vi "equationCalculator.vi"(4 "Time Period":i8, 5 "Max profiles":T1, 6 "startOfTimePeriod":dbl, 7 "derivitave":i8, 8 "aInital (only needed for T0)":dbl, 9 "vInital":dbl, 10 "xInital":dbl, 11 "currentTime":dbl) -> (3 "output variable":dbl)   [LabVIEW 2014]
uses:
  Max profiles.ctl
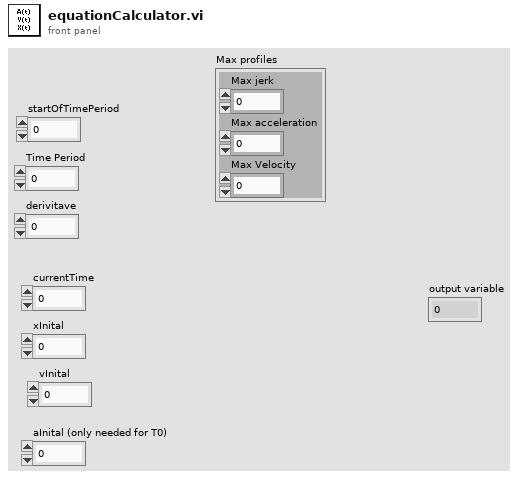
[diagram p1: front panel]
types:
  T1 = typedef "Max profiles.ctl" = cluster{"Max jerk":dbl, "Max acceleration":dbl, "Max Velocity":dbl}
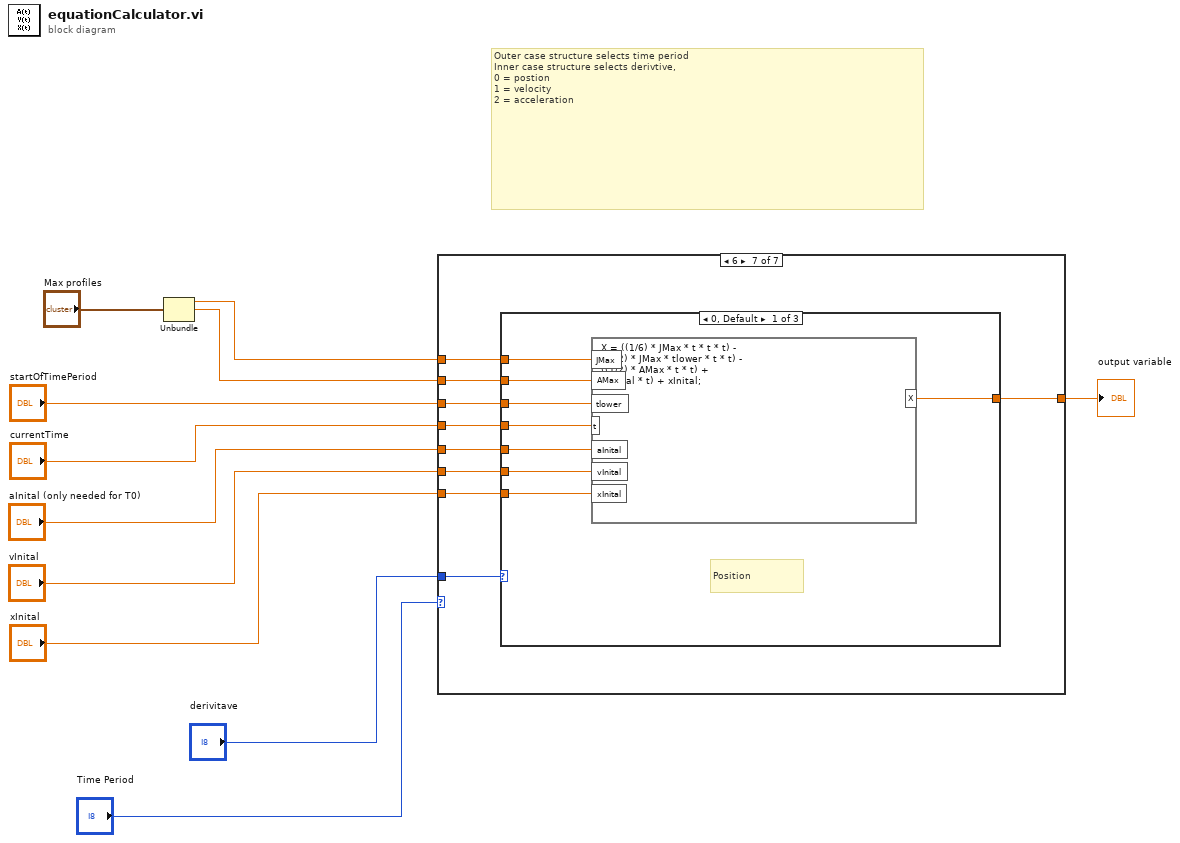
[diagram p0: block diagram]
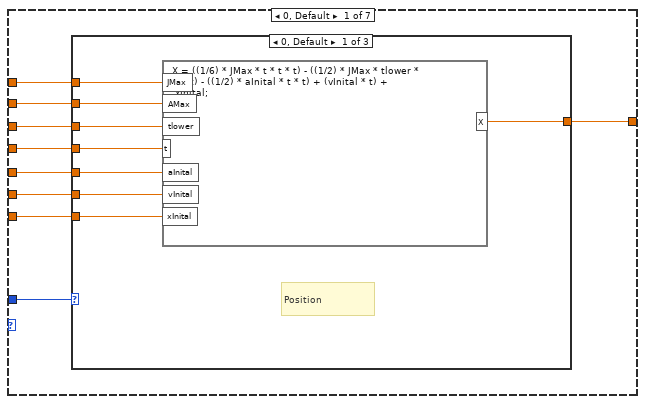
[diagram p2: hidden frame]
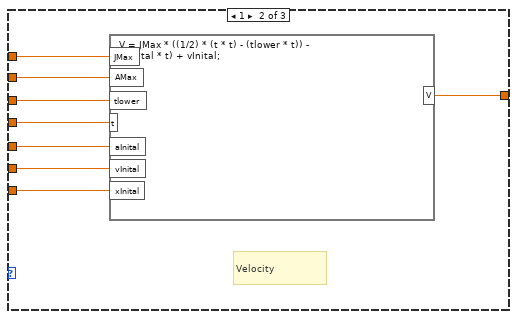
[diagram p3: hidden frame]
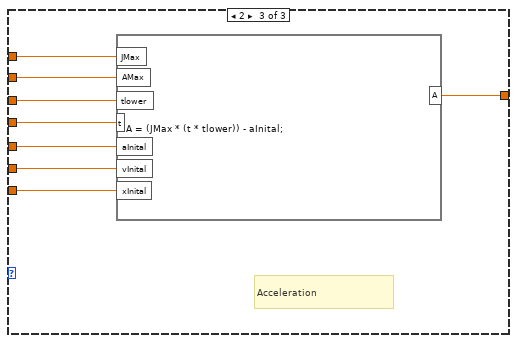
[diagram p4: hidden frame]
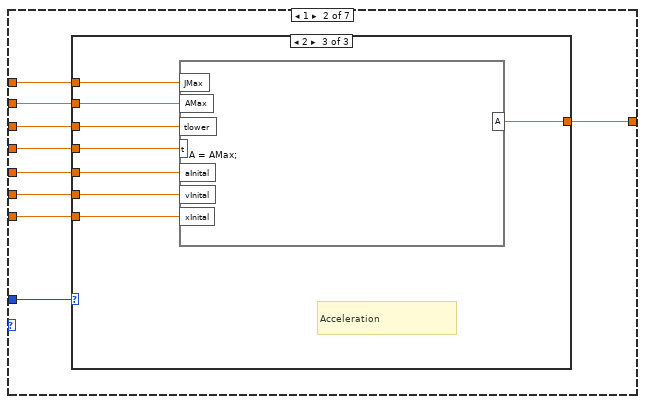
[diagram p5: hidden frame]
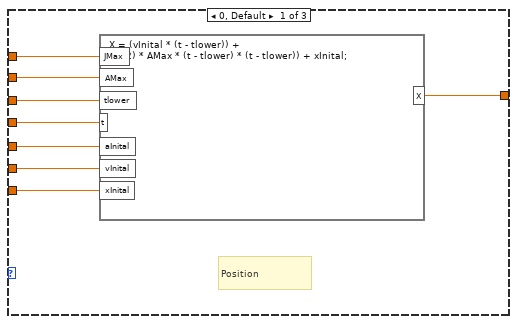
[diagram p6: hidden frame]
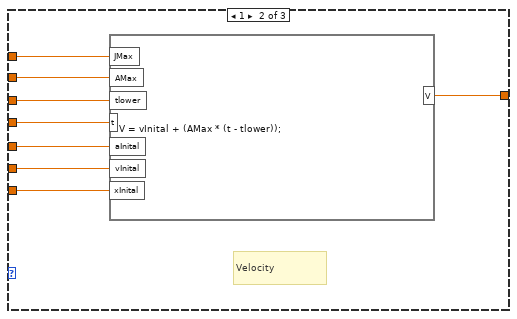
[diagram p7: hidden frame]
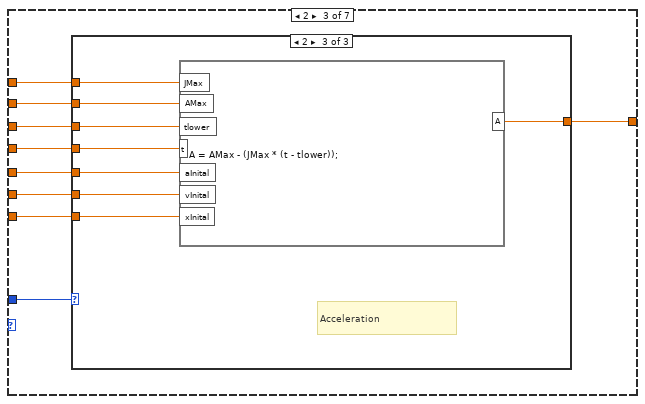
[diagram p8: hidden frame]
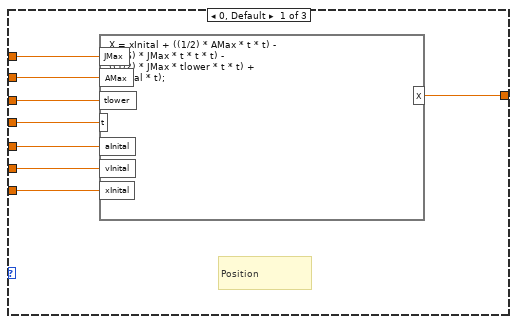
[diagram p9: hidden frame]
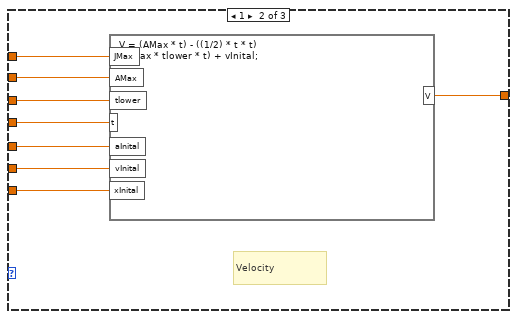
[diagram p10: hidden frame]
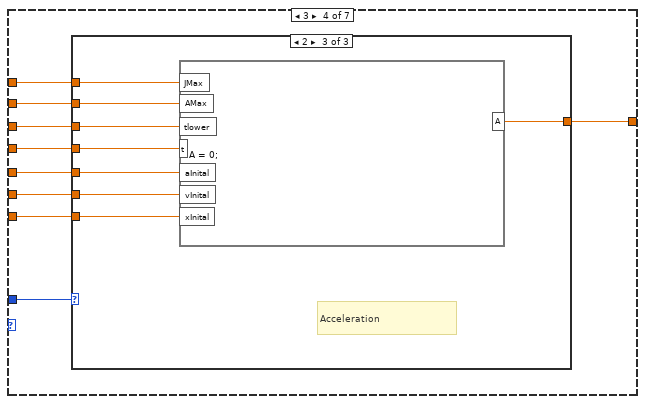
[diagram p11: hidden frame]
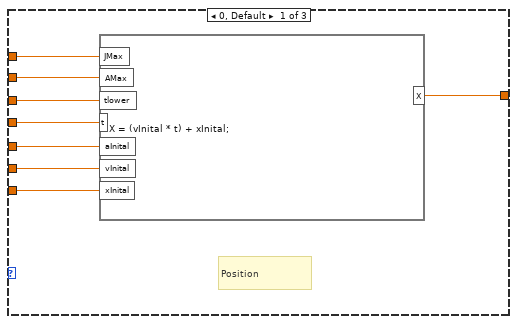
[diagram p12: hidden frame]
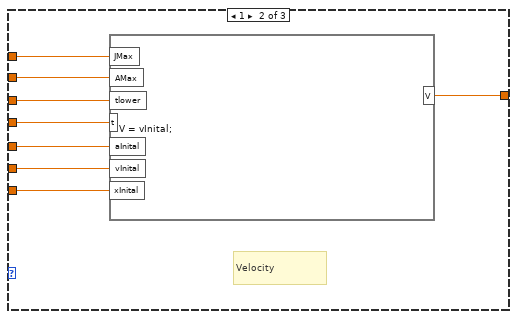
[diagram p13: hidden frame]
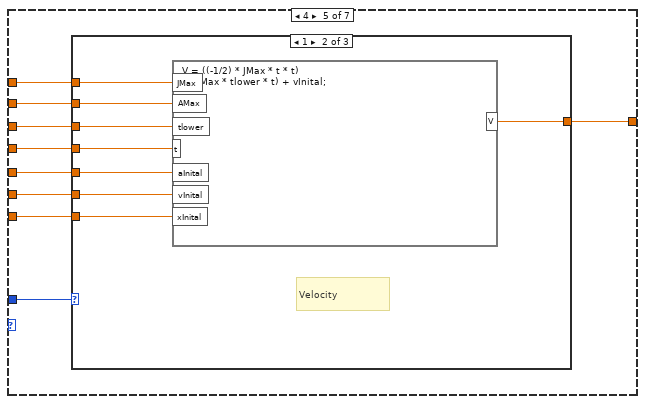
[diagram p14: hidden frame]
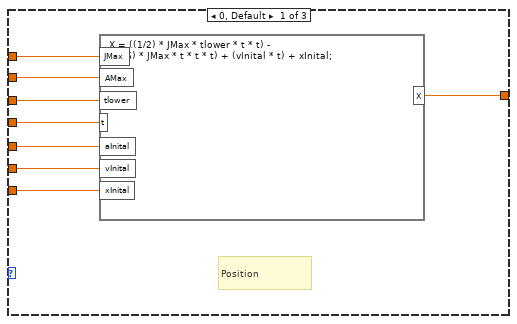
[diagram p15: hidden frame]
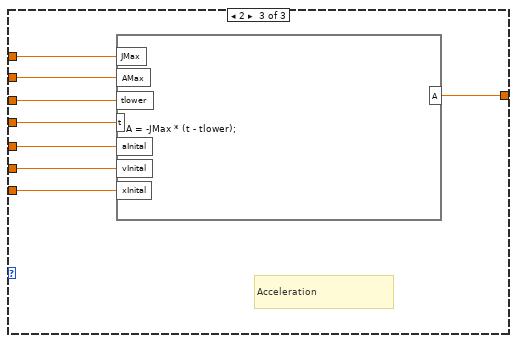
[diagram p16: hidden frame]
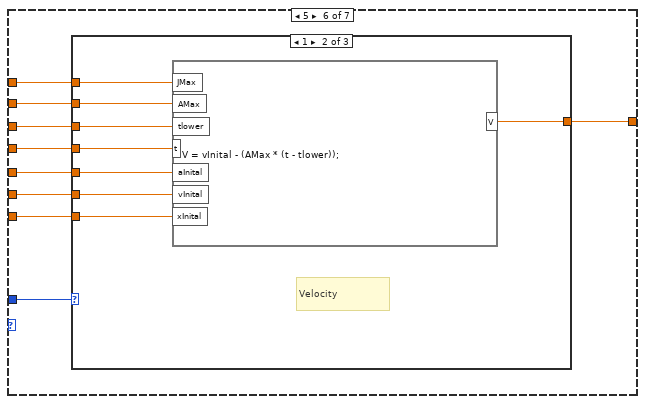
[diagram p17: hidden frame]
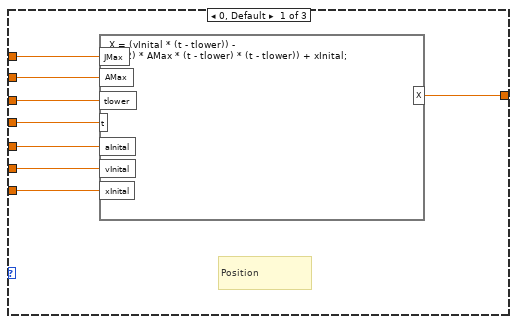
[diagram p18: hidden frame]
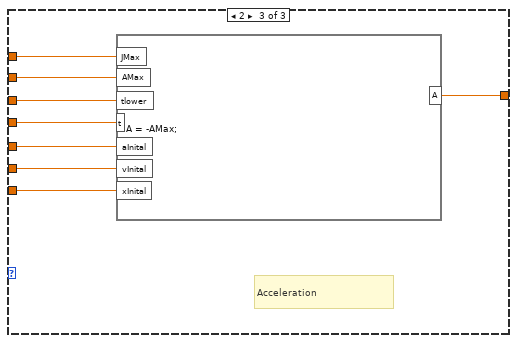
[diagram p19: hidden frame]
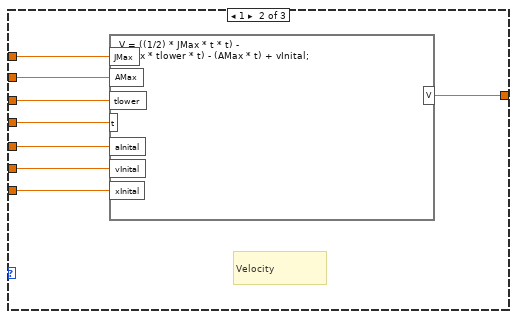
[diagram p20: hidden frame]
diagram:
  # "Outer case structure selects time period\nInner case structure selects derivtive, \n0 = postion\n1 = velocity\n2 = acceleration"
  n1 = Unbundle("Max profiles") -> ("Max jerk"=w2:dbl, "Max acceleration"=w1:dbl)  [unwired: 1 out]
  n2 = case shown="6" "Time Period" {
    tunnel: "derivitave" -> [w20 w53 w86 w119 w152 w185 w218]
    tunnel: w2 -> [w19 w52 w85 w118 w151 w184 w217]
    tunnel: [w18 w51 w84 w117 w150 w183 w216] -> w9
    tunnel: w1 -> [w17 w50 w83 w116 w149 w182 w215]
    tunnel: "startOfTimePeriod" -> [w16 w49 w82 w115 w148 w181 w214]
    tunnel: "currentTime" -> [w15 w48 w81 w114 w147 w180 w213]
    tunnel: "aInital (only needed for T0)" -> [w14 w47 w80 w113 w146 w179 w212]
    tunnel: "vInital" -> [w13 w46 w79 w112 w145 w178 w211]
    tunnel: "xInital" -> [w12 w45 w78 w111 w144 w177 w210]
    frame 0, Default {
      n3 = case shown="0, Default" w20 {
        tunnel: w19 -> [w28 w36 w44]
        tunnel: [w27 w35 w37] -> w18
        tunnel: w17 -> [w26 w34 w43]
        tunnel: w16 -> [w25 w33 w42]
        tunnel: w15 -> [w24 w32 w41]
        tunnel: w14 -> [w23 w31 w40]
        tunnel: w13 -> [w22 w30 w39]
        tunnel: w12 -> [w21 w29 w38]
        frame 0, Default {
          # "Position"
          n4 = formula code="X = ((1/6) * JMax * t * t * t) - ((1/2) * JMax * tlower *\n t * t) - ((1/2) * aInital * t * t) + (vInital * t) +\n xInital;"("JMax"=w28, "t"=w24, "tlower"=w25, "aInital"=w23, "vInital"=w22, "xInital"=w21, "AMax"=w26) -> ("X"=w27:dbl)
        }
        frame 1 {
          # "Velocity"
          n5 = formula code="V = JMax * ((1/2) * (t * t) - (tlower * t)) - \n(aInital * t) + vInital;"("JMax"=w36, "t"=w32, "tlower"=w33, "aInital"=w31, "vInital"=w30, "xInital"=w29, "AMax"=w34) -> ("V"=w35:dbl)
        }
        frame 2 {
          # "Acceleration"
          n6 = formula code="A = (JMax * (t * tlower)) - aInital;"("JMax"=w44, "t"=w41, "tlower"=w42, "aInital"=w40, "vInital"=w39, "xInital"=w38, "AMax"=w43) -> ("A"=w37:dbl)
        }
      }
    }
    frame 1 {
      n7 = case shown="2" w53 {
        tunnel: w52 -> [w61 w69 w77]
        tunnel: [w60 w68 w70] -> w51
        tunnel: w50 -> [w59 w67 w76]
        tunnel: w49 -> [w58 w66 w75]
        tunnel: w48 -> [w57 w65 w74]
        tunnel: w47 -> [w56 w64 w73]
        tunnel: w46 -> [w55 w63 w72]
        tunnel: w45 -> [w54 w62 w71]
        frame 0, Default {
          # "Position"
          n8 = formula code="X = (vInital * (t - tlower)) + \n((1/2) * AMax * (t - tlower) * (t - tlower)) + xInital;"("JMax"=w61, "t"=w57, "tlower"=w58, "aInital"=w56, "vInital"=w55, "xInital"=w54, "AMax"=w59) -> ("X"=w60:dbl)
        }
        frame 1 {
          # "Velocity"
          n9 = formula code="V = vInital + (AMax * (t - tlower));"("JMax"=w69, "t"=w65, "tlower"=w66, "aInital"=w64, "vInital"=w63, "xInital"=w62, "AMax"=w67) -> ("V"=w68:dbl)
        }
        frame 2 {
          # "Acceleration"
          n10 = formula code="A = AMax;"("JMax"=w77, "t"=w74, "tlower"=w75, "aInital"=w73, "vInital"=w72, "xInital"=w71, "AMax"=w76) -> ("A"=w70:dbl)
        }
      }
    }
    frame 2 {
      n11 = case shown="2" w86 {
        tunnel: w85 -> [w94 w102 w110]
        tunnel: [w93 w101 w103] -> w84
        tunnel: w83 -> [w92 w100 w109]
        tunnel: w82 -> [w91 w99 w108]
        tunnel: w81 -> [w90 w98 w107]
        tunnel: w80 -> [w89 w97 w106]
        tunnel: w79 -> [w88 w96 w105]
        tunnel: w78 -> [w87 w95 w104]
        frame 0, Default {
          # "Position"
          n12 = formula code="X = xInital + ((1/2) * AMax * t * t) -\n((1/6) * JMax * t * t * t) -\n((1/2) * JMax * tlower * t * t) +\n(vInital * t);"("JMax"=w94, "t"=w90, "tlower"=w91, "aInital"=w89, "vInital"=w88, "xInital"=w87, "AMax"=w92) -> ("X"=w93:dbl)
        }
        frame 1 {
          # "Velocity"
          n13 = formula code="V = (AMax * t) - ((1/2) * t * t)\n- (JMax * tlower * t) + vInital;"("JMax"=w102, "t"=w98, "tlower"=w99, "aInital"=w97, "vInital"=w96, "xInital"=w95, "AMax"=w100) -> ("V"=w101:dbl)
        }
        frame 2 {
          # "Acceleration"
          n14 = formula code="A = AMax - (JMax * (t - tlower));"("JMax"=w110, "t"=w107, "tlower"=w108, "aInital"=w106, "vInital"=w105, "xInital"=w104, "AMax"=w109) -> ("A"=w103:dbl)
        }
      }
    }
    frame 3 {
      n15 = case shown="2" w119 {
        tunnel: w118 -> [w127 w135 w143]
        tunnel: [w126 w134 w136] -> w117
        tunnel: w116 -> [w125 w133 w142]
        tunnel: w115 -> [w124 w132 w141]
        tunnel: w114 -> [w123 w131 w140]
        tunnel: w113 -> [w122 w130 w139]
        tunnel: w112 -> [w121 w129 w138]
        tunnel: w111 -> [w120 w128 w137]
        frame 0, Default {
          # "Position"
          n16 = formula code="X = (vInital * t) + xInital;"("JMax"=w127, "t"=w123, "tlower"=w124, "aInital"=w122, "vInital"=w121, "xInital"=w120, "AMax"=w125) -> ("X"=w126:dbl)
        }
        frame 1 {
          # "Velocity"
          n17 = formula code="V = vInital;"("JMax"=w135, "t"=w131, "tlower"=w132, "aInital"=w130, "vInital"=w129, "xInital"=w128, "AMax"=w133) -> ("V"=w134:dbl)
        }
        frame 2 {
          # "Acceleration"
          n18 = formula code="A = 0;"("JMax"=w143, "t"=w140, "tlower"=w141, "aInital"=w139, "vInital"=w138, "xInital"=w137, "AMax"=w142) -> ("A"=w136:dbl)
        }
      }
    }
    frame 4 {
      n19 = case shown="1" w152 {
        tunnel: w151 -> [w160 w168 w176]
        tunnel: [w159 w167 w169] -> w150
        tunnel: w149 -> [w158 w166 w175]
        tunnel: w148 -> [w157 w165 w174]
        tunnel: w147 -> [w156 w164 w173]
        tunnel: w146 -> [w155 w163 w172]
        tunnel: w145 -> [w154 w162 w171]
        tunnel: w144 -> [w153 w161 w170]
        frame 0, Default {
          # "Position"
          n20 = formula code="X = ((1/2) * JMax * tlower * t * t) - \n((1/6) * JMax * t * t * t) + (vInital * t) + xInital;"("JMax"=w160, "t"=w156, "tlower"=w157, "aInital"=w155, "vInital"=w154, "xInital"=w153, "AMax"=w158) -> ("X"=w159:dbl)
        }
        frame 1 {
          # "Velocity"
          n21 = formula code="V = ((-1/2) * JMax * t * t) \n+ (JMax * tlower * t) + vInital;"("JMax"=w168, "t"=w164, "tlower"=w165, "aInital"=w163, "vInital"=w162, "xInital"=w161, "AMax"=w166) -> ("V"=w167:dbl)
        }
        frame 2 {
          # "Acceleration"
          n22 = formula code="A = -JMax * (t - tlower);"("JMax"=w176, "t"=w173, "tlower"=w174, "aInital"=w172, "vInital"=w171, "xInital"=w170, "AMax"=w175) -> ("A"=w169:dbl)
        }
      }
    }
    frame 5 {
      n23 = case shown="1" w185 {
        tunnel: w184 -> [w193 w201 w209]
        tunnel: [w192 w200 w202] -> w183
        tunnel: w182 -> [w191 w199 w208]
        tunnel: w181 -> [w190 w198 w207]
        tunnel: w180 -> [w189 w197 w206]
        tunnel: w179 -> [w188 w196 w205]
        tunnel: w178 -> [w187 w195 w204]
        tunnel: w177 -> [w186 w194 w203]
        frame 0, Default {
          # "Position"
          n24 = formula code="X = (vInital * (t - tlower)) - \n((1/2) * AMax * (t - tlower) * (t - tlower)) + xInital;"("JMax"=w193, "t"=w189, "tlower"=w190, "aInital"=w188, "vInital"=w187, "xInital"=w186, "AMax"=w191) -> ("X"=w192:dbl)
        }
        frame 1 {
          # "Velocity"
          n25 = formula code="V = vInital - (AMax * (t - tlower));"("JMax"=w201, "t"=w197, "tlower"=w198, "aInital"=w196, "vInital"=w195, "xInital"=w194, "AMax"=w199) -> ("V"=w200:dbl)
        }
        frame 2 {
          # "Acceleration"
          n26 = formula code="A = -AMax;"("JMax"=w209, "t"=w206, "tlower"=w207, "aInital"=w205, "vInital"=w204, "xInital"=w203, "AMax"=w208) -> ("A"=w202:dbl)
        }
      }
    }
    frame 6 {
      n27 = case shown="0, Default" w218 {
        tunnel: w217 -> [w226 w234 w242]
        tunnel: [w225 w233 w235] -> w216
        tunnel: w215 -> [w224 w232 w241]
        tunnel: w214 -> [w223 w231 w240]
        tunnel: w213 -> [w222 w230 w239]
        tunnel: w212 -> [w221 w229 w238]
        tunnel: w211 -> [w220 w228 w237]
        tunnel: w210 -> [w219 w227 w236]
        frame 0, Default {
          # "Position"
          n28 = formula code="X = ((1/6) * JMax * t * t * t) - \n((1/2) * JMax * tlower * t * t) -\n((1/2) * AMax * t * t) +\n(vInital * t) + xInital;"("JMax"=w226, "t"=w222, "tlower"=w223, "aInital"=w221, "vInital"=w220, "xInital"=w219, "AMax"=w224) -> ("X"=w225:dbl)
        }
        frame 1 {
          # "Velocity"
          n29 = formula code="V = ((1/2) * JMax * t * t) -\n(JMax * tlower * t) - (AMax * t) + vInital;"("JMax"=w234, "t"=w230, "tlower"=w231, "aInital"=w229, "vInital"=w228, "xInital"=w227, "AMax"=w232) -> ("V"=w233:dbl)
        }
        frame 2 {
          # "Acceleration"
          n30 = formula code="A = (JMax * (t - tlower)) - AMax;"("JMax"=w242, "t"=w239, "tlower"=w240, "aInital"=w238, "vInital"=w237, "xInital"=w236, "AMax"=w241) -> ("A"=w235:dbl)
        }
      }
    }
  }
  "output variable" <- w9
